vi "Write Behaviour Tree.vi"(8 "error in (no error)":errorcluster, 10 "BT.lvlib:bt_Node.lvclass":refnum<class "bt_Node.lvclass">, 11 "bt_System in":refnum<class "bt_System.lvclass">) -> (0 "error out":errorcluster, 3 "bt_System out":refnum<class "bt_System.lvclass">)   [LabVIEW 2021, in "BT.lvlib" / "bt_System.lvclass"]
uses:
  bt_System.lvclass
  bt_System.lvclass/bt_System.ctl
  Support/Nodes/abs_Node/bt_Node.lvclass
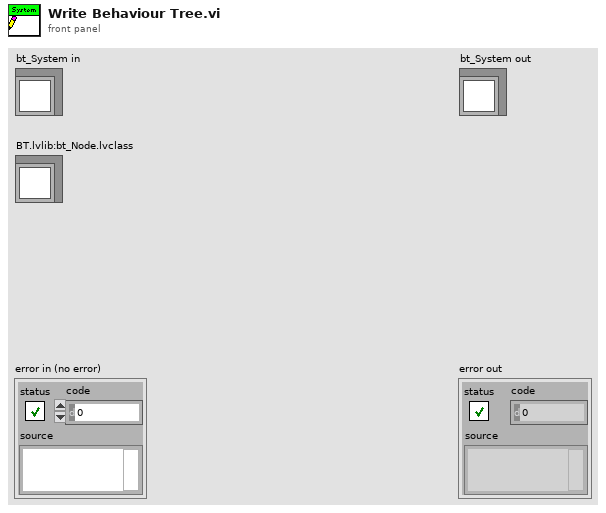
[diagram p1: front panel]
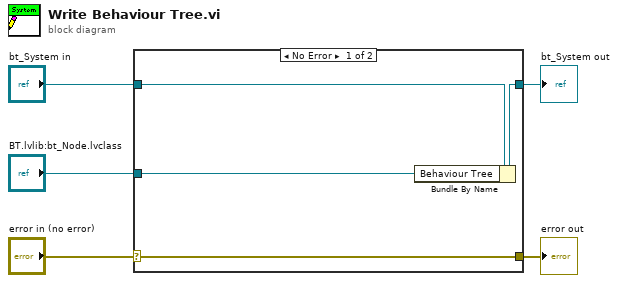
[diagram p0: block diagram]
diagram:
  n1 = case shown="No Error" "error in (no error)" {
    selector: "error in (no error)" -> [w9 w10]
    tunnel: [w9 w10] -> w4
    tunnel: [w7 w11] -> w2
    tunnel: "bt_System in" -> [w8 w11]
    tunnel: "BT.lvlib:bt_Node.lvclass" -> [w6 _]
    frame No Error {
      n2 = Bundle By Name(cluster=w8, "Behaviour Tree"=w6) -> (w7:refnum<class "bt_System.lvclass">)
    }
    frame Error {
    }
  }
  "error out" <- w4
  "bt_System out" <- w2
